vi "Marshall.vi"(8 "error in (no error)":errorcluster, 10 "Variant":variant, 11 "Serializer in":refnum<class "Serializer.lvclass">) -> (0 "error out":errorcluster, 2 "String":string, 3 "Serializer out":refnum<class "Serializer.lvclass">)   [LabVIEW 2013, in "SMOConfig.lvlib" / "Serializer.lvclass"]
uses:
  Serializer.lvclass
  <vilib>/addons/_JKI.lib/Serialization/JSON/JKI JSON Serialization.lvlib
  <vilib>/Utility/VariantDataType/VariantType.lvlib
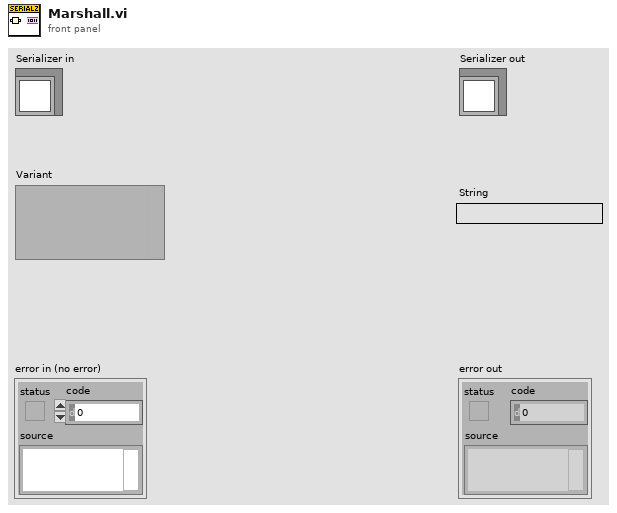
[diagram p1: front panel]
types:
  T1 = typedef "VariantType.lvlib/Type.ctl" = enum8{"Invalid Type", "Void", "I8", "I16", "I32", "I64", "U8", "U16", "U32", "U64", "Single Float", "Double Float", "Extended Float", "Single Complex", "Double Complex", "Extended Complex", "Enum U8", "Enum U16", "Enum U32", "Enum U64", "Single Float With Unit", "Double Float With Unit", "Extended Float With Unit", "Single Complex with Unit", "Double Complex with Unit", "Extended Complex with Unit", "Boolean", "String", "Path", "Picture", "Tag", "Array", "Cluster", "Variant", "LV Variant", "Waveform", "Timestamp", "Digital Waveform", "Digital Data", "ExpressData", "Refnum", "External Data", "VI", "Poly VI", "LabVIEW Class Instance", "Fixed Point"}
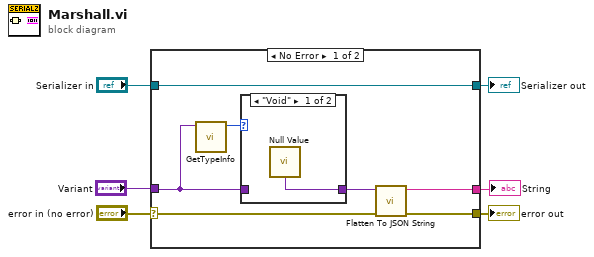
[diagram p0: block diagram]
diagram:
  n1 = case shown="No Error" "error in (no error)" {
    selector: "error in (no error)" -> [w10 w17]
    tunnel: [w11 w17] -> w5
    tunnel: [w13 w16] -> w3
    tunnel: "Serializer in" -> [w13 w16]
    tunnel: "Variant" -> [w8 _]
    tunnel: [w12 _] -> w1
    frame No Error {
      n2 = call <vilib>:"GetTypeInfo.vi"("Variant"=w8) -> ("Type Enum"=w9:T1)  [unwired: 6 in, 4 out]
      n3 = case shown="\"Void\"" w9 {
        tunnel: [w14 w15] -> w7
        tunnel: w8 -> [_ w15]
        frame "Void" {
          n4 = call <vilib>:"Null Value.vi"() -> ("Null"=w14:variant)
        }
        frame Default {
        }
      }
      n5 = call <vilib>:"Flatten To JSON String.vi"("error in (no error)"=w10, "Variant"=w7) -> ("error out"=w11:errorcluster, "JSON String"=w12:string)  [unwired: 8 in]
    }
    frame Error {
    }
  }
  "error out" <- w5
  "Serializer out" <- w3
  "String" <- w1
